vi "Fix offset.vi"(1 "Input":dbl format="%#_13g") -> (0 "Output":dbl format="%#_13g")   [LabVIEW 2018]
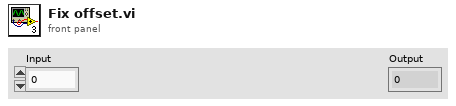
[diagram p1: front panel]
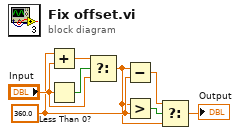
[diagram p0: block diagram]
diagram:
  w4 = 360.0
  n1 = Add(x=w4, y="Input") -> (x+y=w6:dbl)
  n2 = Less Than 0?(x="Input") -> (x < 0?=w8:bool)
  n3 = Select(t=w6, s=w8, f="Input") -> (s? t:f=w3:dbl)
  n4 = Subtract(x=w3, y=w4) -> (x-y=w1:dbl)
  n5 = Greater?(x=w3, y=w4) -> (0:w5:bool)
  n6 = Select(t=w1, s=w5, f=w3) -> (s? t:f=→"Output":dbl)
